vi "Init.vi"(8 "error in (no error)":errorcluster, 10 "Name":string, 11 "BaseResponder in":refnum<class "BaseResponder.lvclass">) -> (0 "error out":errorcluster, 3 "BaseResponder out":refnum<class "BaseResponder.lvclass">)   [LabVIEW 2013, in "BaseResponder.lvclass"]
doc: "Initializes the responder. Call before first use"
uses:
  BaseResponder.lvclass
  BaseResponder.lvclass/BaseResponder.ctl
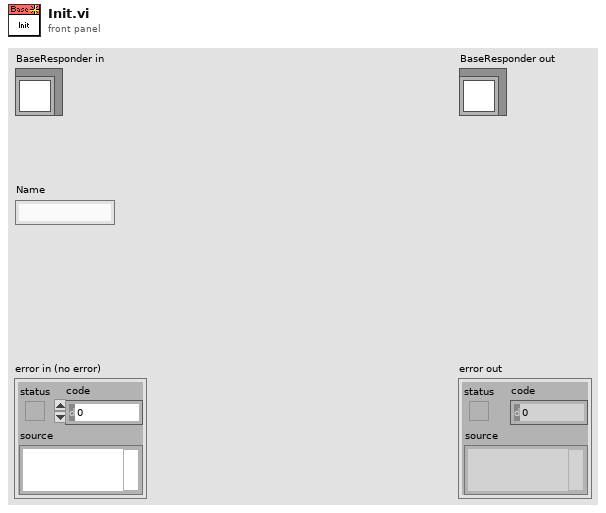
[diagram p1: front panel]
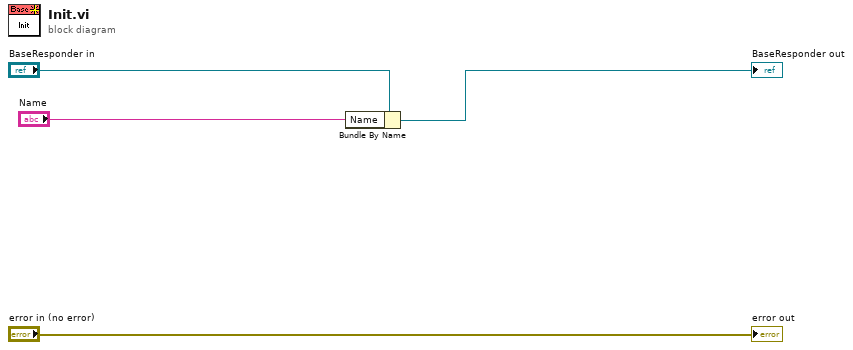
[diagram p0: block diagram]
diagram:
  n1 = Bundle By Name(cluster="BaseResponder in", "Name"="Name") -> (→"BaseResponder out":refnum<class "BaseResponder.lvclass">)
  "error out" <- "error in (no error)"
